vi "Write Group.vi"(8 "error in (no error)":errorcluster, 9 "group values":T1, 10 "id":string, 11 "dsf refnum":T4) -> (0 "error out":errorcluster, 3 "dsf refnum out":T4, 4 "replaced?":bool)   [LabVIEW 2017, in "Data Sharing Framework Core.lvlib" / "Data Sharing Framework Configuration.lvlib"]
doc: "Writes a value to a key in a specified section of the configuration data identified by <B>dsf refnum</B>. This VI modifies data in memory. To write data to disk, use the Close Config Data VI. Wire data to the <B>value</B> input to determine the polymorphic instance to use or manually select the instance."
uses:
  Data Sharing Framework Configuration.lvlib
  Controls/DSF Config Data RefNum.ctl
  Controls/DSF Group Info.ctl
  Controls/DSF Direction.ctl
  Controls/DSF Timing Info.ctl
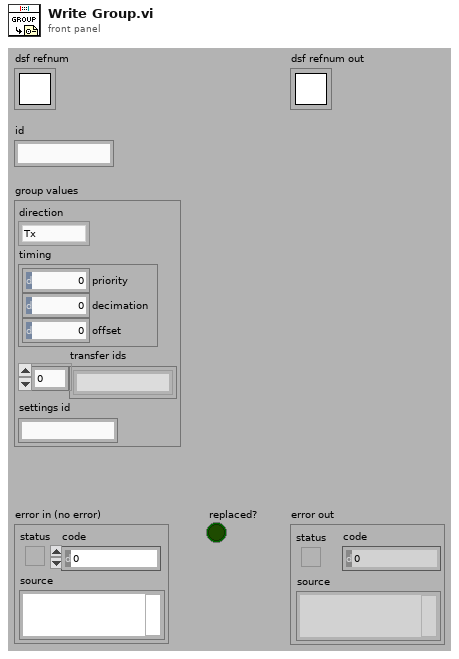
[diagram p1: front panel]
types:
  T1 = typedef "Data Sharing Framework Core.lvlib/Data Sharing Framework Configuration.lvlib/DSF Group Info.ctl" = cluster{"direction":T2, "timing":T3, "transfer ids":string[], "settings id":string}
  T2 = typedef "Data Sharing Framework Core.lvlib/Data Sharing Framework Configuration.lvlib/DSF Direction.ctl" = enum8{"Tx", "Rx"}
  T3 = typedef "Data Sharing Framework Core.lvlib/Data Sharing Framework Configuration.lvlib/DSF Timing Info.ctl" = cluster{"priority":u64, "decimation":u64, "offset":u64}
  T4 = typedef "Data Sharing Framework Core.lvlib/Data Sharing Framework Configuration.lvlib/DSF Config Data RefNum.ctl" = refnum<k1>
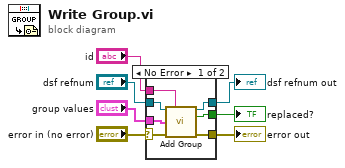
[diagram p0: block diagram]
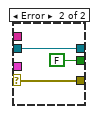
[diagram p2: hidden frame]
diagram:
  n1 = case shown="No Error" "error in (no error)" {
    selector: "error in (no error)" -> [w11 w17]
    tunnel: [w12 w17] -> w6
    tunnel: "id" -> [w14 _]
    tunnel: [w13 FALSE ("key exists?")] -> w4
    tunnel: "dsf refnum" -> [w10 w15]
    tunnel: [w9 w15] -> w2
    tunnel: "group values" -> [w8 _]
    frame No Error {
      n2 = call "Add Group.vi"("dsf refnum"=w10, "id"=w14, "values"=w8, "error in (no error)"=w11) -> ("dsf refnum out"=w9:T4, "exists?"=w13:bool, "error out"=w12:errorcluster)  [unwired: 9 in]
    }
    frame Error {
    }
  }
  "error out" <- w6
  "replaced?" <- w4
  "dsf refnum out" <- w2
